vi "Execute With No Process Model.vi"(9 "Sequence Name":string, 10 "Sequence File To Run":string, 11 "Sequence Context":refnum<k7>) -> (0 "error out":errorcluster)   [LabVIEW 2011]
doc: "Executes a TestStand sequence file with no process model."
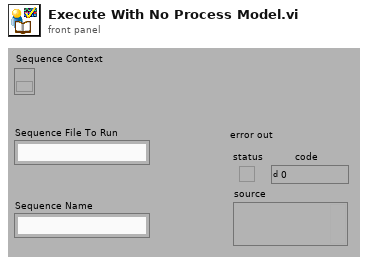
[diagram p1: front panel]
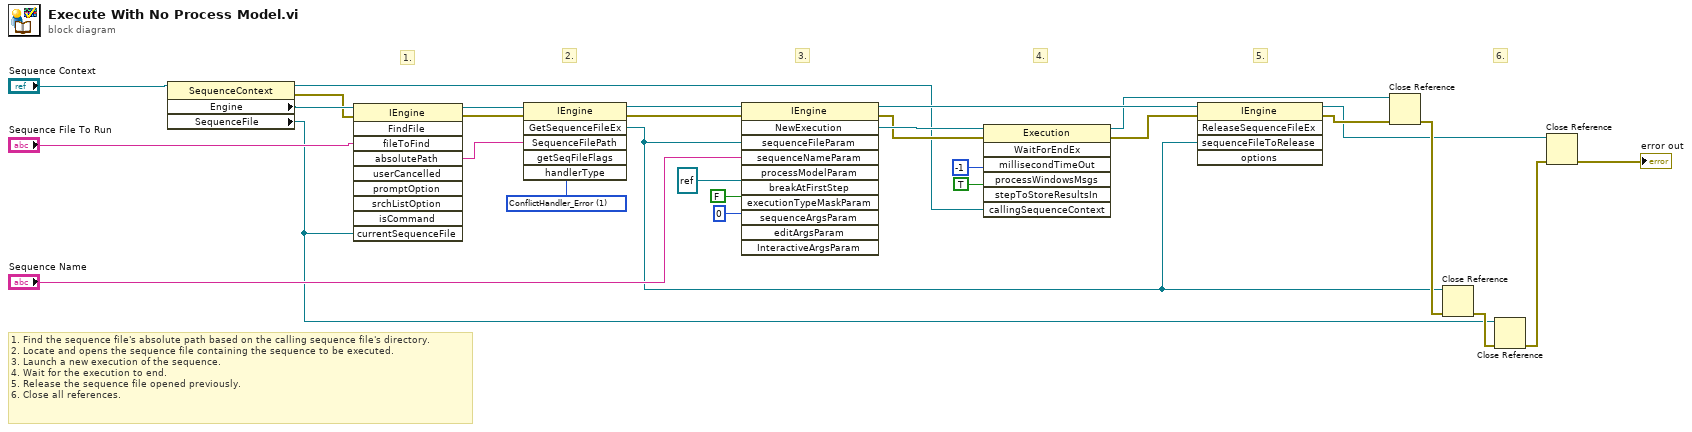
[diagram p0: block diagram]
diagram:
  w30 = 1 items=["ConflictHandler_Error"=1, "ConflictHandler_Prompt"=3, "ConflictHandler_UseGlobalType"=4] ("handlerType")
  # "1."
  # "1. Find the sequence file's absolute path based on the calling sequence file's directory. \n2. Locate and opens the sequence file containing the sequence to be executed.  \n3. Launch a new execution of the sequence.\n4. Wait for the execution to end.\n5. Release the sequence file opened previously.\n6. Close all references."
  # "6."
  # "5."
  # "4."
  # "3."
  # "2."
  n1 = property class="SequenceContext"(reference="Sequence Context") -> (reference out=w16:refnum<k7>, error out=w10:errorcluster, "Engine"=w13:refnum<k7>, "SequenceFile"=w4:refnum<k7>)  [unwired: 1 in]
  n2 = invoke class="IEngine" method="FindFile"(reference=w13, error in=w10, "fileToFind"="Sequence File To Run", "currentSequenceFile"=w4) -> (reference out=w12:refnum<k7>, error out=w11:errorcluster, "absolutePath"=w7:string)  [unwired: 6 in, 7 out]
  n3 = invoke class="IEngine" method="GetSequenceFileEx"(reference=w12, error in=w11, "SequenceFilePath"=w7, "handlerType"=w30) -> (reference out=w29:refnum<k7>, error out=w28:errorcluster, "GetSequenceFileEx"=w3:refnum<k7>)  [unwired: 2 in, 3 out]
  n4 = invoke class="IEngine" method="NewExecution"(reference=w29, error in=w28, "sequenceFileParam"=w3, "sequenceNameParam"="Sequence Name", "processModelParam"=refnum<k7> refnum, "breakAtFirstStep"=FALSE, "executionTypeMaskParam"=0) -> (reference out=w21:refnum<k7>, error out=w24:errorcluster, "NewExecution"=w25:refnum<k7>)  [unwired: 4 in, 8 out]
  n5 = invoke class="Execution" method="WaitForEndEx"(reference=w25, error in=w24, "millisecondTimeOut"=-1, "processWindowsMsgs"=TRUE, "callingSequenceContext"=w16) -> (reference out=w2:refnum<k7>, error out=w20:errorcluster)  [unwired: 2 in, 5 out]
  n6 = invoke class="IEngine" method="ReleaseSequenceFileEx"(reference=w21, error in=w20, "sequenceFileToRelease"=w3) -> (reference out=w5:refnum<k7>, error out=w19:errorcluster)  [unwired: 2 in, 3 out]
  n7 = Close Reference(reference=w2, error in (no error)=w19) -> (error out=w18:errorcluster)
  n8 = Close Reference(reference=w3, error in (no error)=w18) -> (error out=w17:errorcluster)
  n9 = Close Reference(reference=w4, error in (no error)=w17) -> (error out=w6:errorcluster)
  n10 = Close Reference(reference=w5, error in (no error)=w6) -> (error out=→"error out":errorcluster)
